vi "IO Command Error.vi"(4 "error in (no error)":errorcluster, 6 "Command Returned (\"\")":string, 7 "Command Sent (\"\")":string) -> (0 "error out":errorcluster, 3 "HW ERR?":bool)   [LabVIEW 2011]
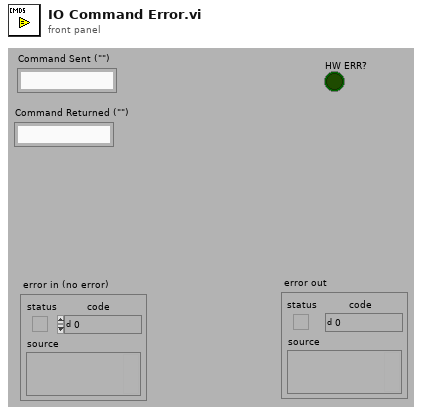
[diagram p1: front panel]
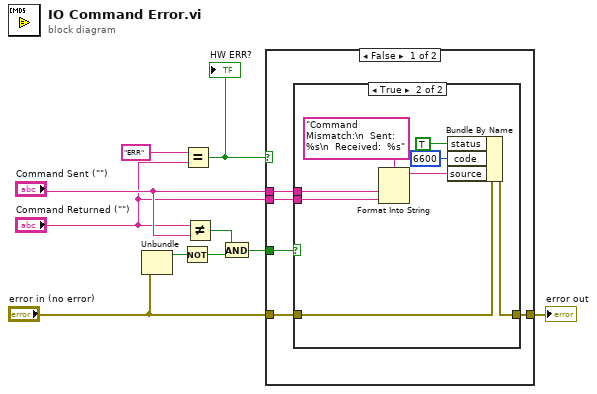
[diagram p0: block diagram]
diagram:
  n1 = Unbundle("error in (no error)") -> ("status"=w8:bool)  [unwired: 2 out]
  n2 = Not(x=w8) -> (.not. x?=w7:bool)
  n3 = Equal?(x="ERR", y="Command Returned (\"\")") -> (x = y?=w1:bool)
  "HW ERR?" <- w1
  n4 = Not Equal?(x="Command Returned (\"\")", y="Command Sent (\"\")") -> (x != y?=w9:bool)
  n5 = And(x=w9, y=w7) -> (x .and. y?=w6:bool)
  n6 = case shown="False" w1 {
    tunnel: "Command Sent (\"\")" -> [w15 _]
    tunnel: w6 -> [w14 _]
    tunnel: "error in (no error)" -> [w13 w25]
    tunnel: [w12 w25] -> w4
    tunnel: "Command Returned (\"\")" -> [w11 _]
    frame False {
      n7 = case shown="True" w14 {
        tunnel: w11 -> [_ w22]
        tunnel: w15 -> [_ w21]
        tunnel: w13 -> [w16 w20]
        tunnel: [w16 w19] -> w12
        frame False {
        }
        frame True {
          n8 = Format Into String(format string="Command Mismatch:\n  Sent:  %s\n  Received:  %s" ("source"), w21, w22) -> (resulting string=w23:string)  [unwired: 2 in, 1 out]
          n9 = Bundle By Name(cluster=w20, "status"=TRUE, "code"=6600, "source"=w23) -> (w19:errorcluster)
        }
      }
    }
    frame True {
    }
  }
  "error out" <- w4
